vi "Listen For Msg.vi"(10 "Address":refnum<data-value>) -> (0 "Error out":errorcluster, 2 "Msg":refnum<class "Msg.lvclass">)   [LabVIEW 2025, in "jettl.lvlib" / "Transport.lvlib" / "Queue.lvlib" / "Queue Transport.lvclass"]
uses:
  Queue Transport.lvclass
  Msg/Msg.lvclass
  Queue Transport.lvclass/Queue Transport.ctl
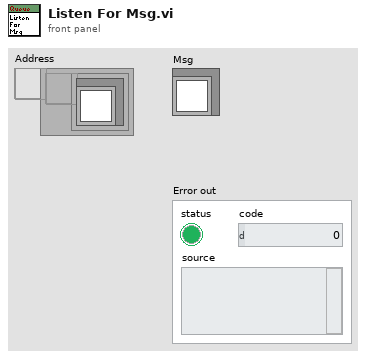
[diagram p1: front panel]
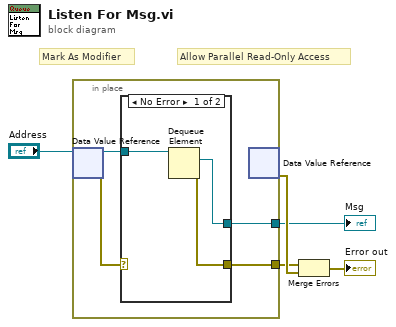
[diagram p0: block diagram]
diagram:
  # "Allow Parallel Read-Only Access"
  # "Mark As Modifier"
  n1 = in-place {
    in-place-border: [w9] -> w4
    in-place-border: [w6] -> w1
    n2 = in-place-dvr #1("Address") -> (w8:refnum<queue>, w7:errorcluster)
    n3 = case shown="No Error" w7 {
      selector: w7 -> [_ w13]
      tunnel: [w11 w13] -> w9
      tunnel: w8 -> [w12 _]
      tunnel: [w10 _] -> w6
      frame No Error {
        n4 = Dequeue Element(queue=w12) -> (element=w10:refnum<class "Msg.lvclass">, error out=w11:errorcluster)  [unwired: 2 in, 2 out]
      }
      frame Error {
      }
    }
    n5 = in-place-dvr #1() -> (w5:errorcluster)  [unwired: 1 in, 1 out]
  }
  "Msg" <- w1
  n6 = Merge Errors(w4, w5) -> (→"Error out":errorcluster)
